vi "thermo_clear.vi"(8 "error in (no error)":errorcluster, 11 "thermo in":T1={"type"=enum."COMET Tx5xx (ethernet)", "comment"="", "tag"="", "refresh"=0.0, "IP"="", "port"=0, "VISA"="", "last readout"=timestamp(0 s since 1904-01-01), "TCP ref"=refnum, "VISA sess"="", "idn"="", "press"=0.0, "RH"=0.0, "temp"=0.0, "pres cor"=[], "RH cor"=[], "temp cor"=[], "try left"=0, "failed"=FALSE, "RTD set"=[], "RTD inv"=[], "range"=0.0, "net mode"=enum."MODBUS", "try fail"=enum."Stop trying - return NaN", "timeout [s]"=0.0, "max retries"=0, "sim t [deg]"=0.0} {"RTD inv" format="%.1f"; "RTD set" format="%.1f"; "temp cor" format="%.1f"; "RH cor" format="%.1f"; "pres cor" format="%.1f"; "refresh" min=0.1 max=1000.0 format="%.2f"}) -> (0 "error out":errorcluster, 3 "thermo out":T1={"type"=enum."COMET Tx5xx (ethernet)", "comment"="", "tag"="", "refresh"=0.0, "IP"="", "port"=0, "VISA"="", "last readout"=timestamp(0 s since 1904-01-01), "TCP ref"=refnum, "VISA sess"="", "idn"="", "press"=0.0, "RH"=0.0, "temp"=0.0, "pres cor"=[], "RH cor"=[], "temp cor"=[], "try left"=0, "failed"=FALSE, "RTD set"=[], "RTD inv"=[], "range"=0.0, "net mode"=enum."MODBUS", "try fail"=enum."Stop trying - return NaN", "timeout [s]"=0.0, "max retries"=0, "sim t [deg]"=0.0} {"RTD inv" format="%.1f"; "RTD set" format="%.1f"; "temp cor" format="%.1f"; "RH cor" format="%.1f"; "pres cor" format="%.1f"; "refresh" min=0.1 max=1000.0 format="%.2f"})   [LabVIEW 2020]
uses:
  thermo.ctl
  thermo_types.ctl
  Thermometer Fail Action.ctl
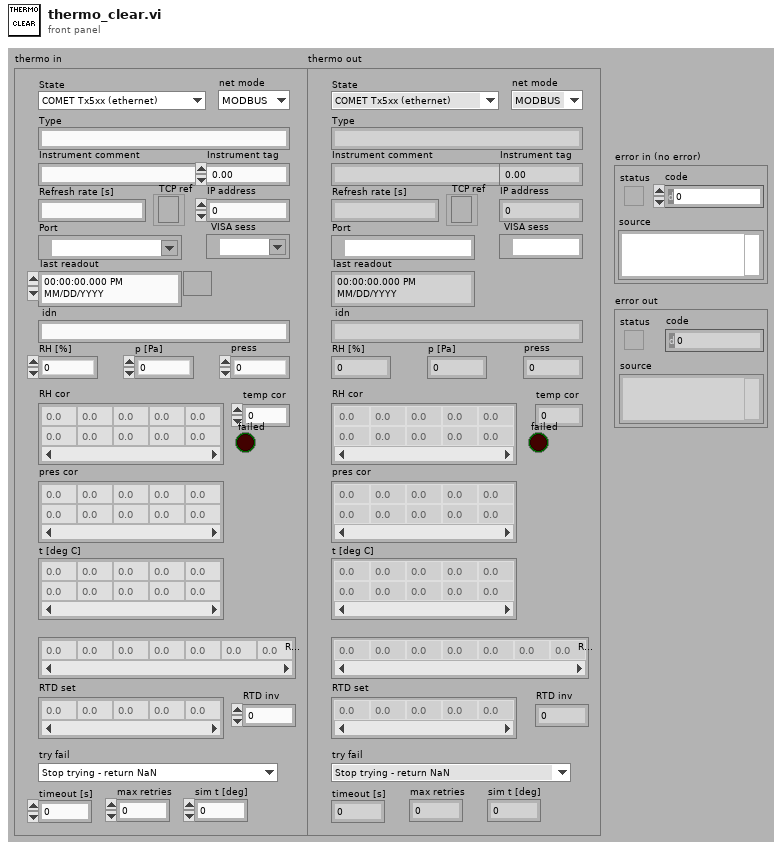
[diagram p1: front panel]
types:
  T1 = typedef "thermo.ctl" = cluster{"type":T2, "comment":string, "tag":string, "refresh":dbl, "IP":string, "port":u16, "VISA":refnum<visa-resource-name>, "last readout":timestamp, "TCP ref":refnum<k5>, "VISA sess":refnum<visa-resource-name>, "idn":string, "press":dbl, "RH":dbl, "temp":dbl, "pres cor":dbl[][], "RH cor":dbl[][], "temp cor":dbl[][], "try left":i32, "failed":bool, "RTD set":dbl[], "RTD inv":dbl[], "range":dbl, "net mode":enum16{"MODBUS", "HTTP"}, "try fail":T3, "timeout [s]":dbl, "max retries":i32, "sim t [deg]":dbl}
  T2 = typedef "thermo_types.ctl" = enum16{"Disabled", "Simulated", "COMET Tx5xx (ethernet)", "Keithley 2002 (GPIB) + RTD", "Agilent 344xx (GPIB) + RTD"}
  T3 = typedef "Thermometer Fail Action.ctl" = enum16{"Stop trying - keep last value", "Stop trying - return NaN", "Generate error - stop sweep"}
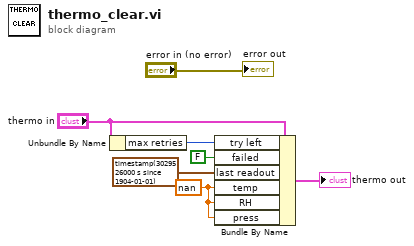
[diagram p0: block diagram]
diagram:
  w4 = nan ("temp")
  n1 = Unbundle By Name("thermo in") -> ("max retries"=w1:i32)
  n2 = Bundle By Name(cluster="thermo in", "try left"=w1, "failed"=FALSE, "last readout"=timestamp(3029526000 s since 1904-01-01), "temp"=w4, "RH"=w4, "press"=w4) -> (→"thermo out":T1)
  "error out" <- "error in (no error)"
